vi "RX JESD.vi"(0 "rxjesd.control":T1) -> (4 "trigger output enable":bool, 6 "trigger value":bool)   [LabVIEW 2019]
uses:
  <vilib>/rvi/eio/common/nirviEmuTemplateMethod_errors.vi
  <vilib>/eio/EIONode/EIONode.xnode
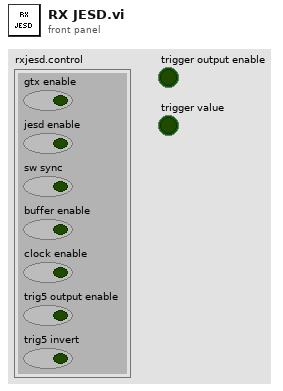
[diagram p1: front panel]
types:
  T1 = cluster{"gtx enable":bool, "jesd enable":bool, "sw sync":bool, "buffer enable":bool, "clock enable":bool, "trig5 output enable":bool, "trig5 invert":bool}
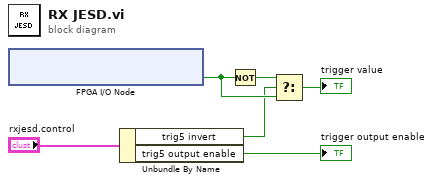
[diagram p0: block diagram]
diagram:
  n1 = xnode "FPGA I/O Node"() -> ("7902R IO Socket\\aSyncToPin"=w5:bool)  [unwired: 1 in, 1 out]
  n2 = Unbundle By Name("rxjesd.control") -> ("trig5 invert"=w3:bool, "trig5 output enable"=→"trigger output enable":bool)
  n3 = Not(x=w5) -> (.not. x?=w6:bool)
  n4 = Select(t=w6, s=w3, f=w5) -> (s? t:f=→"trigger value":bool)
